vi "关键参数组合 (子VI).vi"(9 "table":string="3090仪器参数", 10 "因子编码":string, 11 "data":string[](array[string])) -> (3 "字符串":string)   [LabVIEW 2016, in "数据传输系统-04.lvlib"]
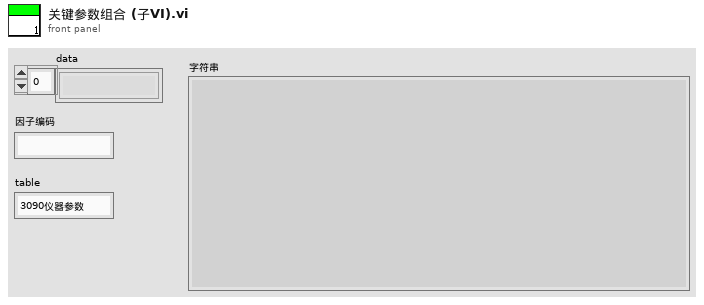
[diagram p1: front panel]
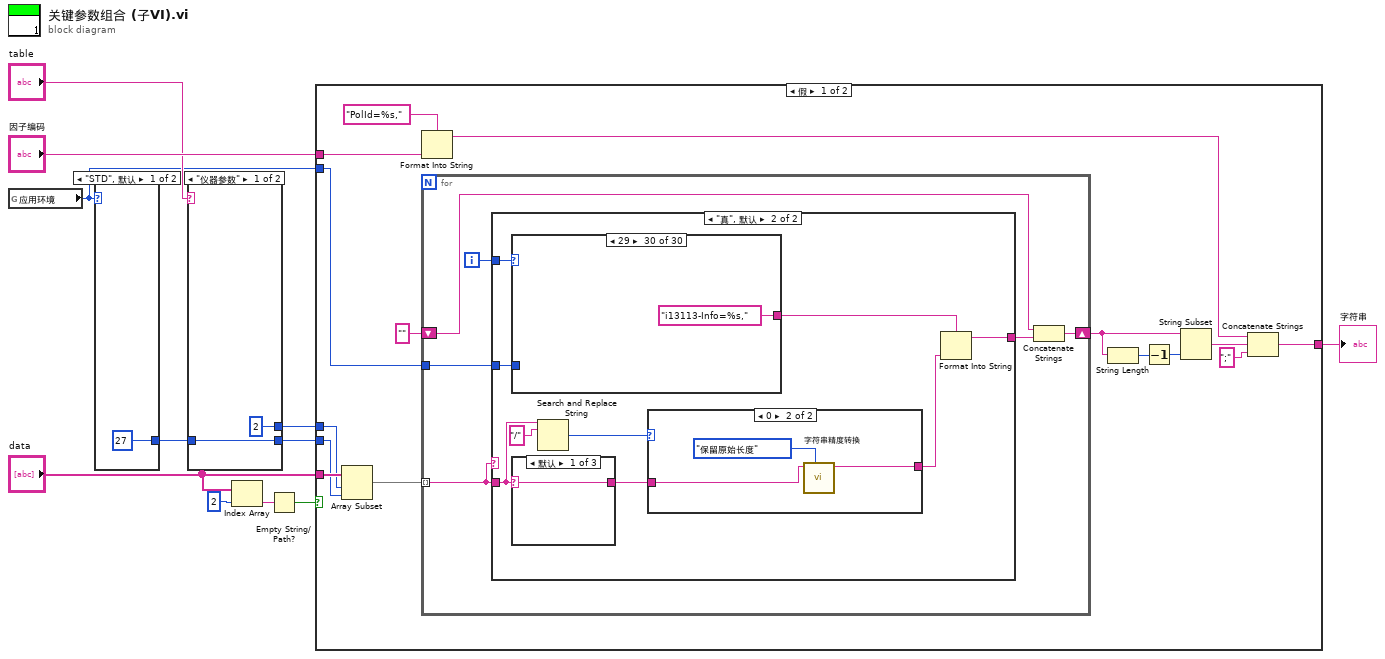
[diagram p0: block diagram]
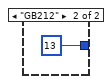
[diagram p2: hidden frame]
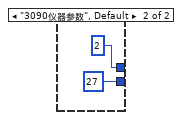
[diagram p3: hidden frame]
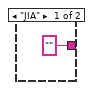
[diagram p4: hidden frame]
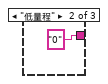
[diagram p5: hidden frame]
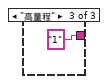
[diagram p6: hidden frame]
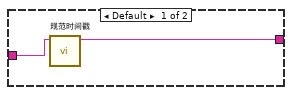
[diagram p7: hidden frame]
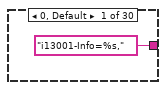
[diagram p8: hidden frame]
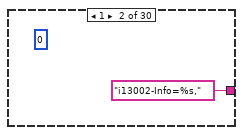
[diagram p9: hidden frame]
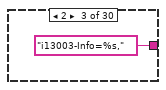
[diagram p10: hidden frame]
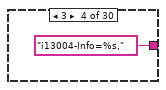
[diagram p11: hidden frame]
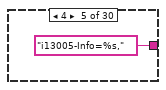
[diagram p12: hidden frame]
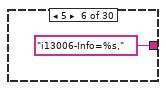
[diagram p13: hidden frame]
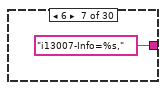
[diagram p14: hidden frame]
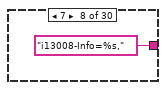
[diagram p15: hidden frame]
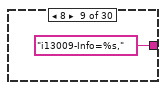
[diagram p16: hidden frame]
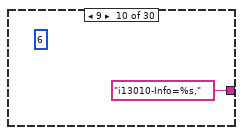
[diagram p17: hidden frame]
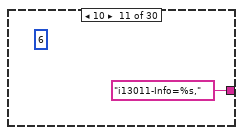
[diagram p18: hidden frame]
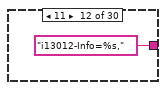
[diagram p19: hidden frame]
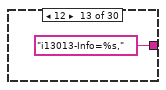
[diagram p20: hidden frame]
diagram:
  n1 = global read "断电保存全局.vi" "应用环境"() -> (w3:enum16{"STD", "GB212"})
  n2 = case shown="\"STD\", 默认" w3 {
    tunnel: [27 ("长度") 13 ("长度")] -> w2
    frame "STD", Default {
    }
    frame "GB212" {
    }
  }
  n3 = case shown="\"仪器参数\"" "table" {
    tunnel: [w14 27 ("长度")] -> w5
    tunnel: [2 ("索引") 2 ("索引")] -> w4
    tunnel: w2 -> [w14 _]
    frame "仪器参数" {
    }
    frame "3090仪器参数", Default {
    }
  }
  n4 = Index Array(array="data", index=2 ("索引")) -> (element=w10:string)
  n5 = Empty String/Path?(string/path=w10) -> (empty?=w9:bool)
  n6 = case shown="假" w9 {
    tunnel: [w31 ""] -> w8
    tunnel: "data" -> [w30 _]
    tunnel: "因子编码" -> [w27 _]
    tunnel: w5 -> [w25 _]
    tunnel: w4 -> [w19 _]
    tunnel: w3 -> [w18 _]
    frame False {
      n7 = Array Subset(array=w30, index=w19, length=w25) -> (w29:string[])
      n8 = Format Into String(format string="PolId=%s,", w27) -> (resulting string=w26:string)  [unwired: 2 in, 1 out]
      n9 = for {
        shift-right: [w35] -> w21
        shift-left: "" -> [w37]
        tunnel: w29 -> [w34] mode=indexing
        tunnel: w18 -> [w33]
        i -> [w38]
        n10 = case shown="\"真\", 默认" w34 {
          tunnel: w38 -> [_ w48]
          tunnel: ["" w46] -> w36
          tunnel: w34 -> [_ w41]
          tunnel: w33 -> [_ w42]
          frame "JIA" {
          }
          frame "真", Default {
            n11 = case shown="29" w48 {
              tunnel: ["i13001-Info=%s," "i13002-Info=%s," "i13003-Info=%s," "i13004-Info=%s," "i13005-Info=%s," "i13006-Info=%s," "i13007-Info=%s," "i13008-Info=%s," "i13009-Info=%s," "i13010-Info=%s," "i13011-Info=%s," "i13012-Info=%s," "i13013-Info=%s," w71 "i13015-Info=%s," "i13016-Info=%s," "i13017-Info=%s," "i13101-Info=%s," "i13102-Info=%s," "i13103-Info=%s," "i13104-Info=%s," "i13105-Info=%s," "i13106-Info=%s," "i13107-Info=%s," "i13108-Info=%s," "i13109-Info=%s," "i13110-Info=%s," "i13111-Info=%s," "i13112-Info=%s," "i13113-Info=%s,"] -> w47
              tunnel: w42 -> [_ _ _ _ _ _ _ _ _ _ _ _ _ w70 _ _ _ _ _ _ _ _ _ _ _ _ _ _ _ _]
              frame 0, Default {
              }
              frame 1 {
                (unwired) 0 ("数据精度")
              }
              frame 2 {
              }
              frame 3 {
              }
              frame 4 {
              }
              frame 5 {
              }
              frame 6 {
              }
              frame 7 {
              }
              frame 8 {
              }
              frame 9 {
                (unwired) 6 ("数据精度")
              }
              frame 10 {
                (unwired) 6 ("数据精度")
              }
              frame 11 {
              }
              frame 12 {
              }
              frame 13 {
                n12 = case shown="\"GB212\"" w70 {
                  tunnel: ["i13110-Info=%s," "i13014-Info=%s,"] -> w71
                  frame "STD", Default {
                  }
                  frame "GB212" {
                  }
                }
              }
              frame 14 {
              }
              frame 15 {
              }
              frame 16 {
              }
              frame 17 {
              }
              frame 18 {
              }
              frame 19 {
              }
              frame 20 {
              }
              frame 21 {
              }
              frame 22 {
              }
              frame 23 {
              }
              frame 24 {
              }
              frame 25 {
              }
              frame 26 {
              }
              frame 27 {
              }
              frame 28 {
              }
              frame 29 {
              }
            }
            n13 = case shown="默认" w41 {
              selector: w41 -> [w49 _ _]
              tunnel: [w49 "0" "1"] -> w40
              frame Default {
              }
              frame "低量程" {
              }
              frame "高量程" {
              }
            }
            n14 = Search and Replace String(input string=w41, search string="/" ("搜索字符串")) -> (number of replacements=w45:i32)  [unwired: 6 in, 3 out]
            n15 = case shown="0" w45 {
              tunnel: w40 -> [w53 w56]
              tunnel: [w52 w55] -> w43
              frame Default {
                n16 = call "规范时间戳.vi"("字符串"=w53) -> ("result string"=w52:string)  [unwired: 10 in]
              }
              frame 0 {
                n17 = call "字符串精度转换.vi"("枚举"=enum16{"小数位修约", "保留原始长度"}."保留原始长度", "输入字符串"=w56) -> ("输出字符串"=w55:string)  [unwired: 8 in, 1 out]
              }
            }
            n18 = Format Into String(format string=w47, w43) -> (resulting string=w46:string)  [unwired: 2 in, 1 out]
          }
        }
        n19 = Concatenate Strings(w37, w36) -> (w35:string)
      }
      n20 = String Length(string=w21) -> (length=w22:i32)
      n21 = Decrement(x=w22) -> (x-1=w23:i32)
      n22 = String Subset(string=w21, length (rest)=w23) -> (substring=w20:string)  [unwired: 1 in]
      n23 = Concatenate Strings(w26, w20, ";" ("字符串")) -> (w31:string)
    }
    frame True {
    }
  }
  "字符串" <- w8
